vi "Dynamixel Function mapping.vi"(2 "data In":i32, 3 "GenericDriveCommand":T2="DePowerMotor") -> (0 "data Out":u32, 1 "Function":T1)   [LabVIEW 2022 SP3]
uses:
  Traverses/~subVIs/GenericDriveCommand.ctl
  Dynamixel Commands.ctl
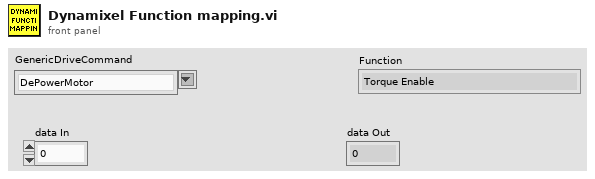
[diagram p1: front panel]
types:
  T1 = typedef "Dynamixel Commands.ctl" = enum16{"Torque Enable", "Present Position", "Threshold", "Max Position Limit", "Acceleration Profile", "Velocity Profile", "Goal Position", "Position Proportional Gain", "Position Integral Gain", "Position Differential Gain ", "Shutdown", "Write Operating Mode", "Read Operating Mode"}
  T2 = typedef "GenericDriveCommand.ctl" = string
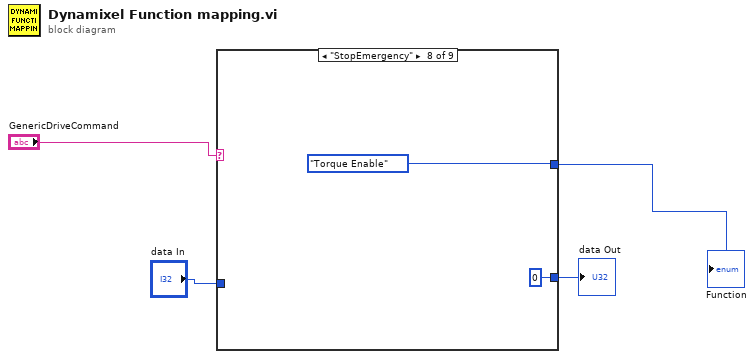
[diagram p0: block diagram]
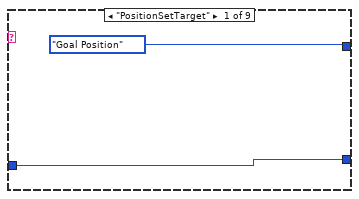
[diagram p2: hidden frame]
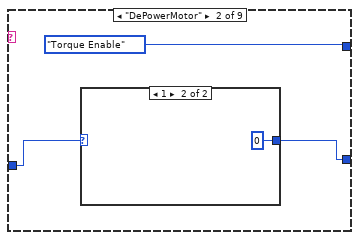
[diagram p3: hidden frame]
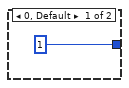
[diagram p4: hidden frame]
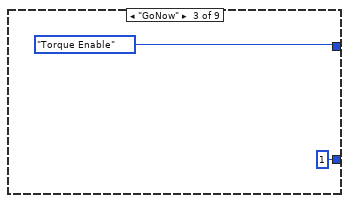
[diagram p5: hidden frame]
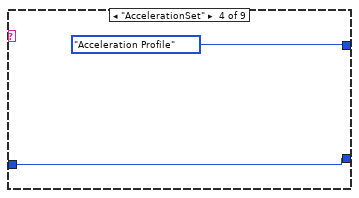
[diagram p6: hidden frame]
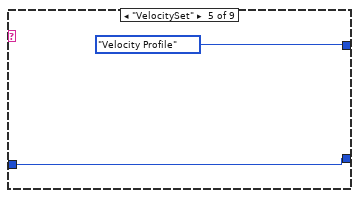
[diagram p7: hidden frame]
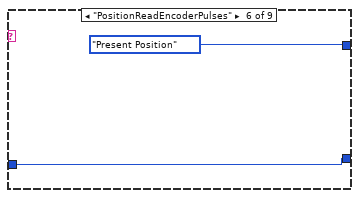
[diagram p8: hidden frame]
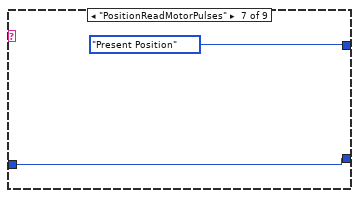
[diagram p9: hidden frame]
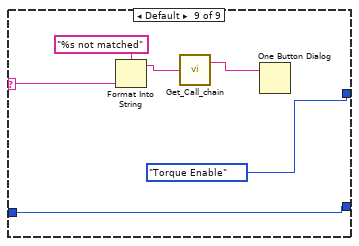
[diagram p10: hidden frame]
diagram:
  n1 = case shown="\"StopEmergency\"" "GenericDriveCommand" {
    selector: "GenericDriveCommand" -> [_ _ _ _ _ _ _ _ w28]
    tunnel: [Dynamixel_Commands."Goal Position" ("Function") Dynamixel_Commands."Torque Enable" ("Function") Dynamixel_Commands."Torque Enable" ("Function") Dynamixel_Commands."Acceleration Profile" ("Function") Dynamixel_Commands."Velocity Profile" ("Function") Dynamixel_Commands."Present Position" ("Function") Dynamixel_Commands."Present Position" ("Function") Dynamixel_Commands."Torque Enable" ("Function") Dynamixel_Commands."Torque Enable" ("Function")] -> w3
    tunnel: [w5 w7 u32 1 ("data In") w14 w16 w18 w20 u32 0 ("data In") w26] -> w2
    tunnel: "data In" -> [w5 w8 _ w14 w16 w18 w20 _ w26]
    frame "PositionSetTarget" {
    }
    frame "DePowerMotor" {
      n2 = case shown="1" w8 {
        tunnel: [u32 1 ("data In") u32 0 ("data In")] -> w7
        frame 0, Default {
        }
        frame 1 {
        }
      }
    }
    frame "GoNow" {
    }
    frame "AccelerationSet" {
    }
    frame "VelocitySet" {
    }
    frame "PositionReadEncoderPulses" {
    }
    frame "PositionReadMotorPulses" {
    }
    frame "StopEmergency" {
    }
    frame Default {
      n3 = Format Into String(format string="%s not matched", w28) -> (resulting string=w25:string)  [unwired: 2 in, 1 out]
      n4 = call "Get_Call_chain.vi"("Message"=w25) -> ("Output String"=w24:string)  [unwired: 1 out]
      n5 = One Button Dialog(message=w24) -> ()  [unwired: 1 in, 1 out]
    }
  }
  "Function" <- w3
  "data Out" <- w2
